vi "Clousure.vi"(8 "error in (no error)":errorcluster, 11 "EnchantedRoom":refnum<class "EnchantedRoom.lvclass">) -> (0 "error out":errorcluster, 3 "EnchantedRoom":refnum<class "EnchantedRoom.lvclass">)   [LabVIEW 2020, in "EnchantedRoom.lvclass"]
uses:
  EnchantedRoom.lvclass
  Room/Room.lvclass
  EnchantedRoom.lvclass/EnchantedRoom.ctl
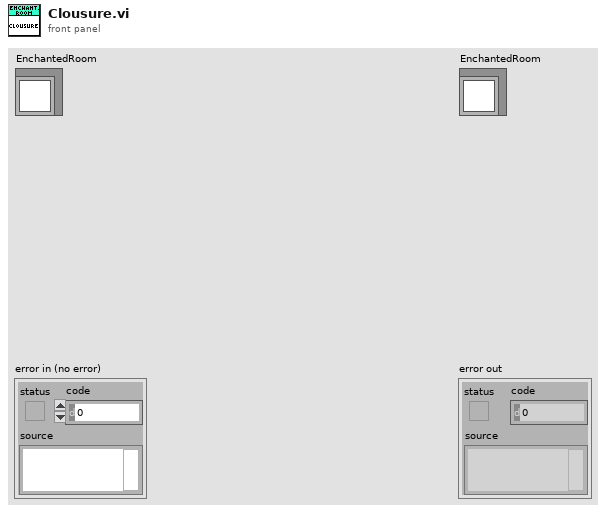
[diagram p1: front panel]
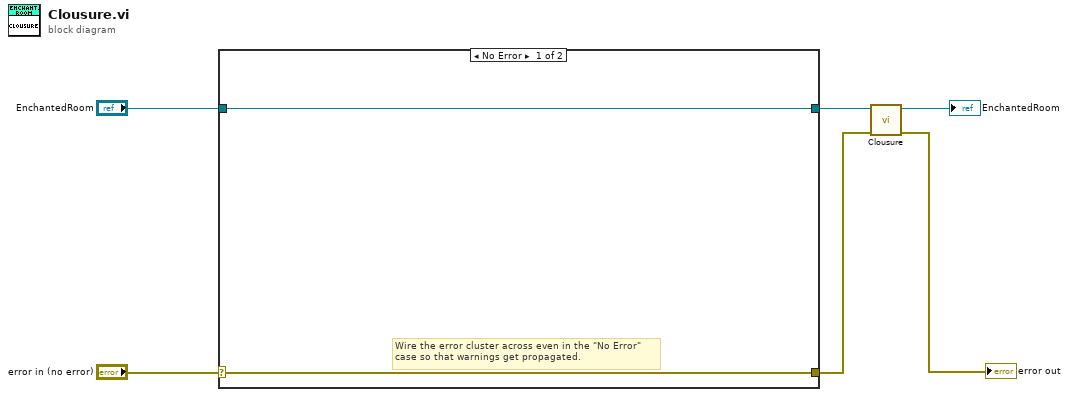
[diagram p0: block diagram]
diagram:
  n1 = case shown="No Error" "error in (no error)" {
    selector: "error in (no error)" -> [w7 w10]
    tunnel: [w7 w10] -> w2
    tunnel: [w8 w9] -> w4
    tunnel: "EnchantedRoom" -> [w8 w9]
    frame No Error {
      # "Wire the error cluster across even in the \"No Error\"\ncase so that warnings get propagated."
    }
    frame Error {
    }
  }
  n2 = call-parent "Clousure.vi"("error in (no error)"=w2, "Room"=w4) -> ("error out"=→"error out":errorcluster, "Room"=→"EnchantedRoom":refnum<class "EnchantedRoom.lvclass">)  [unwired: 8 in]
